vi "Esophageal_GenerateSubfolders_CommandFiles.vi"(8 "error in":errorcluster, 10 "Command File Location":path=path "C:/Users/ABGS_/Desktop/ABGS_RT_HRME Frames/CNN_RealTime/20201129/YNetDeploy/CommandFiles/LabVIEW/cmds.json", 11 "Patient Data Folder":path=path "C:/Users/ABGS_/Desktop/ABGS_RT_HRME Frames/TestFolders") -> (0 "error out":errorcluster, 1 "Rep Image Path":path, 2 "HRME Scores":path, 3 "HRME Path":path)   [LabVIEW 2021]
panel:
  out "JSON string":string
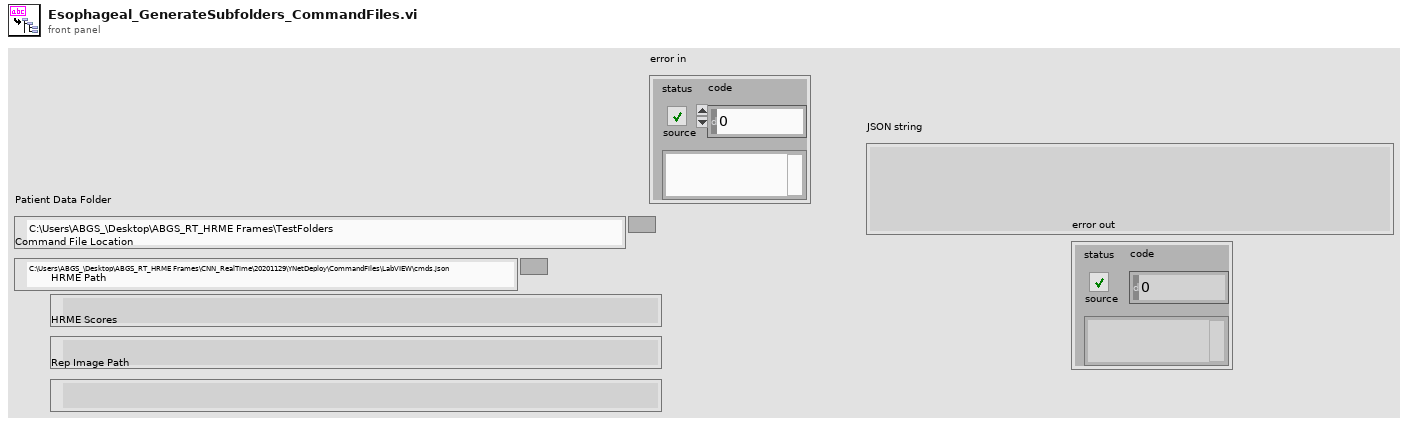
[diagram p1: front panel]
types:
  T1 = cluster{"Source":string, "Destination":string, "CMD":string, "Time":string}
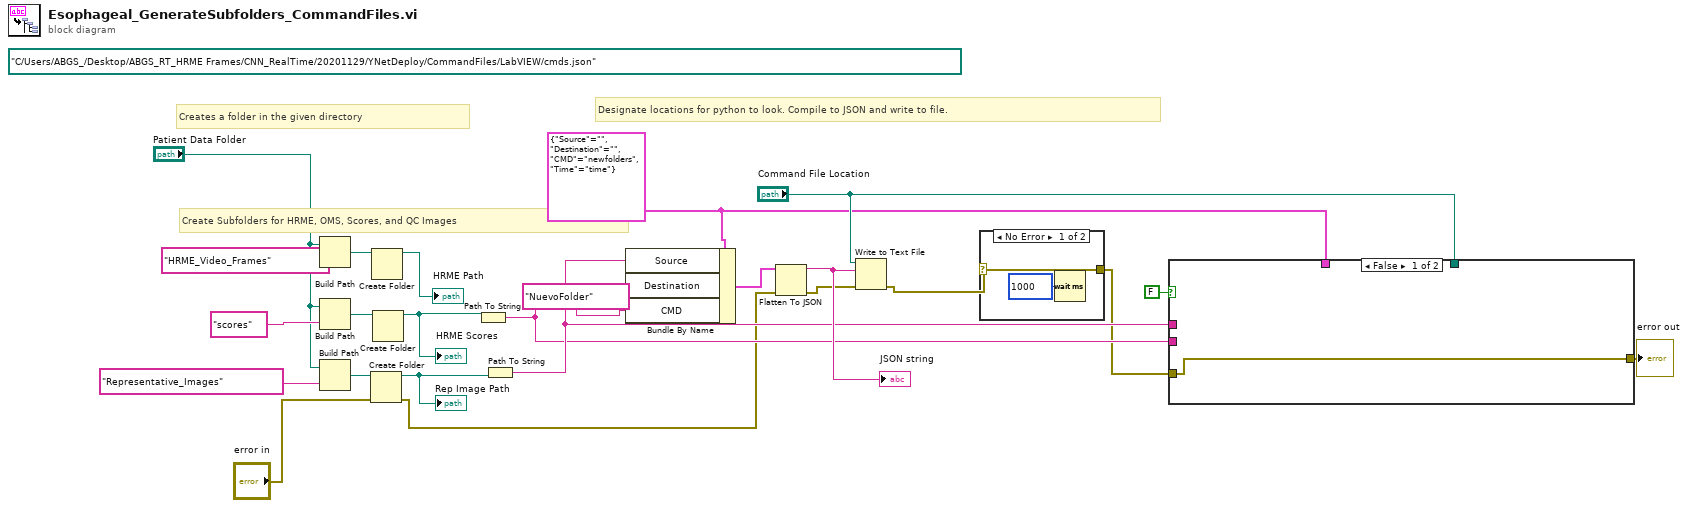
[diagram p0: block diagram]
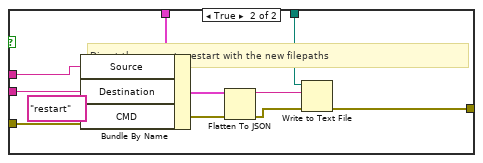
[diagram p2: hidden frame]
diagram:
  (unwired) path "C:/Users/ABGS_/Desktop/ABGS_RT_HRME Frames/CNN_RealTime/20201129/YNetDeploy/CommandFiles/LabVIEW/cmds.json" ("Command File Location")
  w9 = T1 {"Source"="", "Destination"="", "CMD"="newfolders", "Time"="time"} ("Output JSON File")
  # "Designate locations for python to look. Compile to JSON and write to file."
  # "Create Subfolders for HRME, OMS, Scores, and QC Images"
  # "Creates a folder in the given directory"
  n1 = Build Path(base path="Patient Data Folder", name or relative path="HRME_Video_Frames") -> (appended path=w22:path)
  n2 = Build Path(base path="Patient Data Folder", name or relative path="scores") -> (appended path=w21:path)
  n3 = Build Path(base path="Patient Data Folder", name or relative path="Representative_Images") -> (appended path=w20:path)
  n4 = Create Folder(path (use dialog)=w20, error in="error in") -> (created path=w1:path, error out=w4:errorcluster)  [unwired: 1 in, 1 out]
  "Rep Image Path" <- w1
  n5 = Create Folder(path (use dialog)=w22) -> (created path=→"HRME Path":path)  [unwired: 2 in, 2 out]
  n6 = Create Folder(path (use dialog)=w21) -> (created path=w17:path)  [unwired: 2 in, 2 out]
  "HRME Scores" <- w17
  n7 = Path To String(path=w17) -> (string=w11:string)
  n8 = Path To String(path=w1) -> (string=w12:string)
  n9 = Bundle By Name(cluster=w9, "Source"=w12, "Destination"=w11, "CMD"="NuevoFolder") -> (w15:T1)
  n10 = Flatten To JSON(anything=w15, error in (no error)=w4) -> (JSON string=w14:string, 11:w13:errorcluster)  [unwired: 1 in]
  "JSON string" <- w14
  n11 = Write to Text File(file (use dialog)="Command File Location", text=w14, error in=w13) -> (error out=w8:errorcluster)  [unwired: 1 in, 2 out]
  n12 = case shown="No Error" w8 {
    selector: w8 -> [w26 w27]
    tunnel: [w26 w27] -> w7
    frame No Error {
      n13 = Wait (ms)(milliseconds to wait=u32 1000) -> ()  [unwired: 1 out]
    }
    frame Error {
    }
  }
  n14 = case shown="False" FALSE {
    tunnel: w12 -> [_ w37]
    tunnel: w11 -> [_ w36]
    tunnel: "Command File Location" -> [_ w33]
    tunnel: w9 -> [_ w31]
    tunnel: w7 -> [w28 w30]
    tunnel: [w28 w29] -> w3
    frame False {
    }
    frame True {
      # "Direct the queue to restart with the new filepaths"
      n15 = Bundle By Name(cluster=w31, "Source"=w37, "Destination"=w36, "CMD"="restart") -> (w35:T1)
      n16 = Flatten To JSON(anything=w35, error in (no error)=w30) -> (JSON string=w34:string, 11:w32:errorcluster)  [unwired: 1 in]
      n17 = Write to Text File(file (use dialog)=w33, text=w34, error in=w32) -> (error out=w29:errorcluster)  [unwired: 1 in, 2 out]
    }
  }
  "error out" <- w3
